vi "LC Language Global.vi"(7 "Mode":T1, 8 "error in (no error)":errorcluster caption="Error In", 10 "String In":string) -> (0 "error out":errorcluster caption="Error Out", 3 "Read":T2)   [LabVIEW 2020]
uses:
  LC Language Global.ctl
  LC Global Mode.ctl
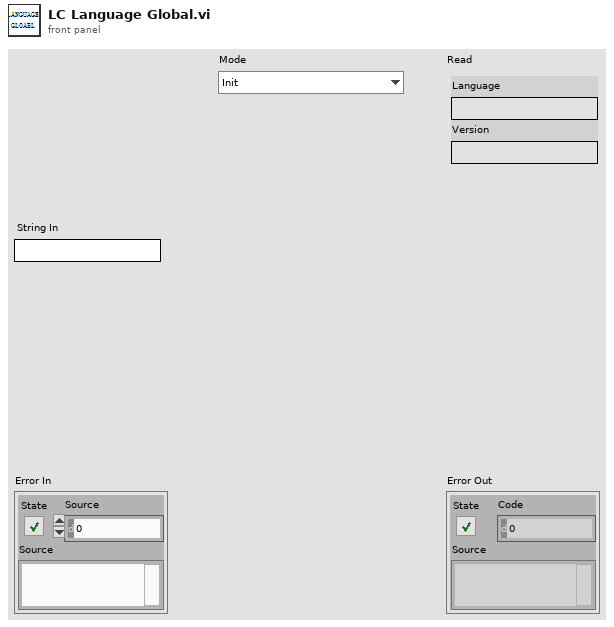
[diagram p1: front panel]
types:
  T1 = typedef "LC Global Mode.ctl" = enum16{"Init", "Read", "Write Language", "Write Version", "Save"}
  T2 = typedef "LC Language Global.ctl" = cluster{"Language":string, "Version":string}
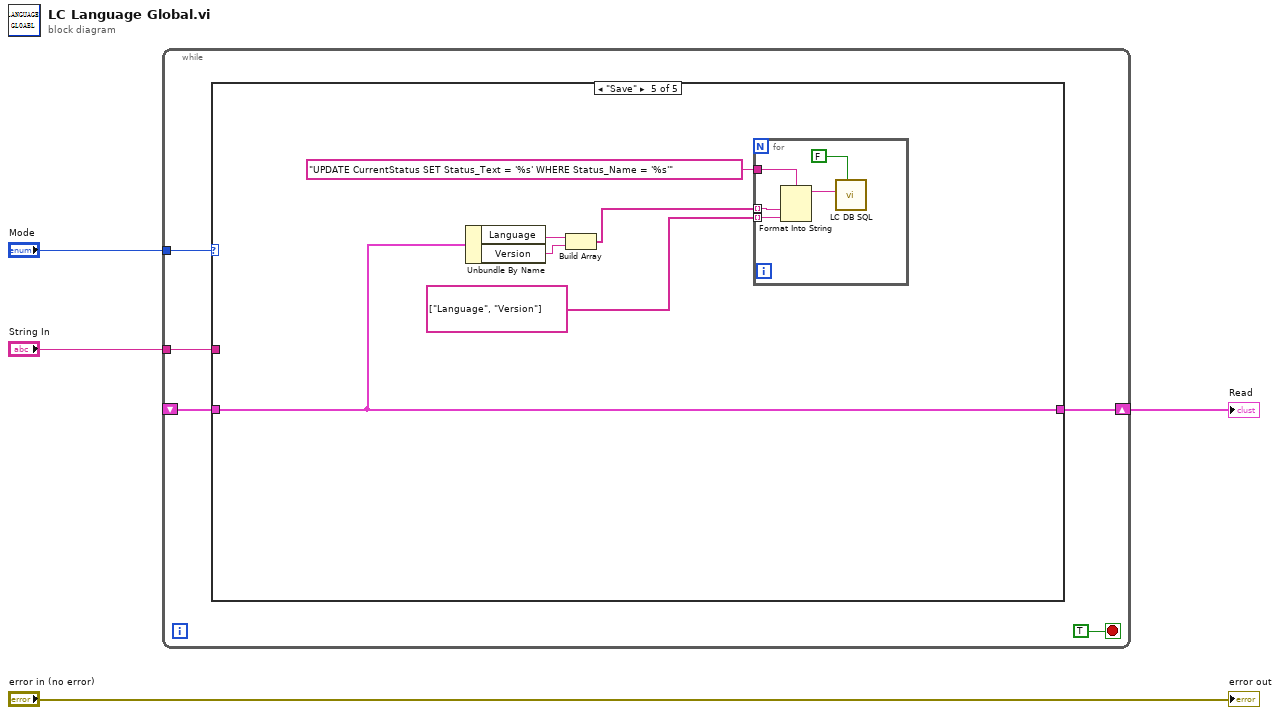
[diagram p0: block diagram]
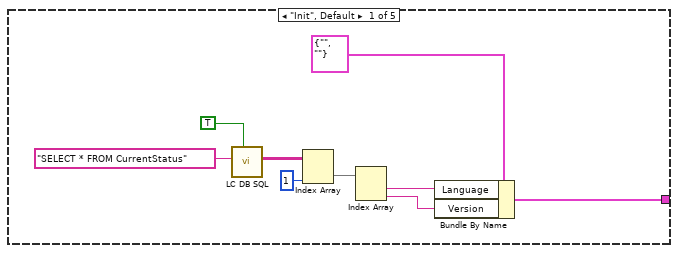
[diagram p2: hidden frame]
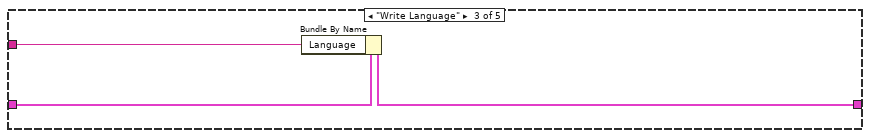
[diagram p4: hidden frame]
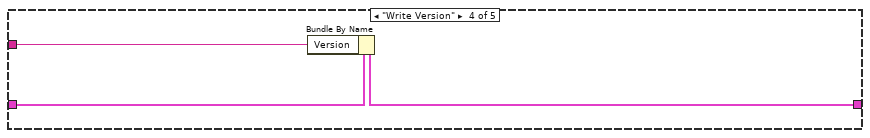
[diagram p5: hidden frame]
diagram:
  n1 = while {
    tunnel: "Mode" -> [w9]
    shift-right: [w7] -> w4
    shift-left: _ -> [w6]
    tunnel: "String In" -> [w5]
    stop <- TRUE stop-if-true
    n2 = case shown="\"Save\"" w9 {
      tunnel: [w12 w19 w20 w23 w31] -> w7
      tunnel: w6 -> [_ w19 w22 w25 w31]
      tunnel: w5 -> [_ _ w21 w24 _]
      frame "Init", Default {
        n3 = call "LC DB SQL.vi"("Get Record"=TRUE ("Read?"), "SQL query"="SELECT * FROM CurrentStatus") -> ("Record"=w15:string[][])  [unwired: 7 in, 2 out]
        n4 = Index Array(array=w15, index (col)=1 ("禁用的索引 (列)")) -> (element=w13:string[])  [unwired: 1 in]
        n5 = Index Array(array=w13) -> (element #1=w11:string, element #2=w10:string)  [unwired: 2 in]
        n6 = Bundle By Name(cluster=T2 {"Language"="", "Version"=""} ("Write"), "Language"=w11, "Version"=w10) -> (w12:T2)
      }
      frame "Read" {
      }
      frame "Write Language" {
        n7 = Bundle By Name(cluster=w22, "Language"=w21) -> (w20:T2)
      }
      frame "Write Version" {
        n8 = Bundle By Name(cluster=w25, "Version"=w24) -> (w23:T2)
      }
      frame "Save" {
        n9 = Unbundle By Name(w31) -> ("Language"=w30:string, "Version"=w29:string)
        n10 = Build Array(w30, w29) -> (w26:string[])
        n11 = for {
          tunnel: "UPDATE CurrentStatus SET Status_Text = '%s' WHERE Status_Name = '%s'" ("SQL query") -> [w36]
          tunnel: string[] ["Language", "Version"] -> [w35] mode=indexing
          tunnel: w26 -> [w34] mode=indexing
          n12 = Format Into String(format string=w36, w34, w35) -> (resulting string=w33:string)  [unwired: 2 in, 1 out]
          n13 = call "LC DB SQL.vi"("Get Record"=FALSE, "SQL query"=w33) -> ()  [unwired: 7 in, 3 out]
        }
      }
    }
  }
  "Read" <- w4
  "error out" <- "error in (no error)"
